vi "Write Global Locked.vi"(8 "error in (no error)":errorcluster, 10 "Global":refnum<class "System.lvclass">, 11 "Shifter in":refnum<class "Shifter.lvclass">) -> (0 "error out":errorcluster, 3 "Shifter out":refnum<class "Shifter.lvclass">)   [LabVIEW 2013, in "Shifter.lvclass"]
uses:
  Shifter.lvclass
  System/System.lvclass
  Robot Global Data.vi
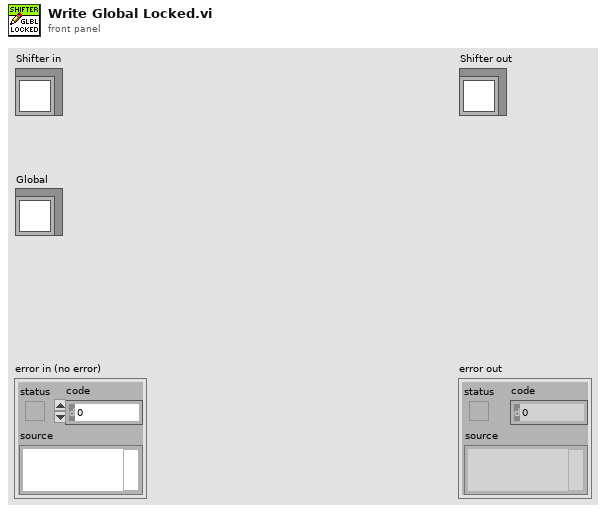
[diagram p1: front panel]
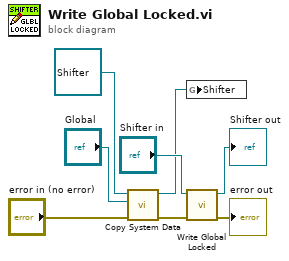
[diagram p0: block diagram]
diagram:
  n1 = call "Copy System Data.vi"("error in (no error)"="error in (no error)", "System Original"="Global", "System in"=refnum<class "Shifter.lvclass"> refnum ("Shifter.lvclass")) -> ("error out"=w2:errorcluster, "System out"=w1:refnum<class "Shifter.lvclass">)  [unwired: 7 in]
  n2 = global write "Robot Global Data.vi" "Shifter"(w1) -> ()
  n3 = call-parent "Write Global Locked.vi"("error in (no error)"=w2, "System in"="Shifter in") -> ("error out"=→"error out":errorcluster, "System out"=→"Shifter out":refnum<class "Shifter.lvclass">)  [unwired: 8 in]
